vi "DSF.Engine.Plugin.Set Engine Base Pointer.vi"(8 "error in (no error)":errorcluster, 10 "Engine Base Pointer":refnum<class "DSF.Engine.Pointer.DBL.lvclass">, 11 "Plugin in":refnum<class "DSF.Engine.Plugin.lvclass">) -> (0 "error out":errorcluster, 3 "Plugin out":refnum<class "DSF.Engine.Plugin.lvclass">)   [LabVIEW 2017, in "DSF.Engine.lvlib" / "DSF.Engine.Plugin.lvclass"]
uses:
  DSF.Engine.Plugin.lvclass
  Pointer/DSF.Engine.Pointer.DBL.lvclass
  DSF.Engine.Plugin.lvclass/DSF.Engine.Plugin.ctl
  Transfer/DSF.Engine.Transfer Group.lvclass
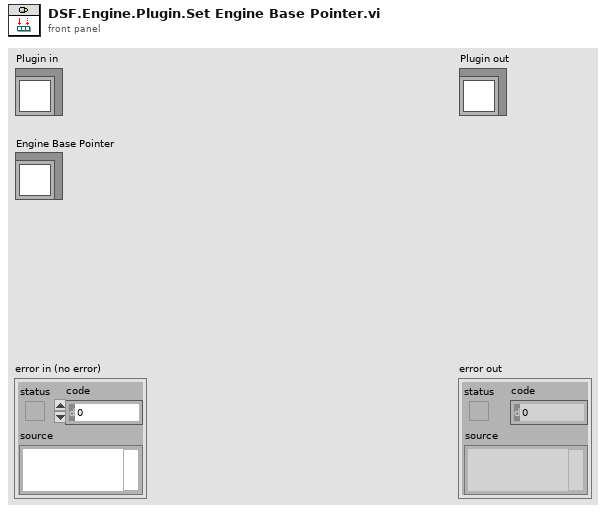
[diagram p1: front panel]
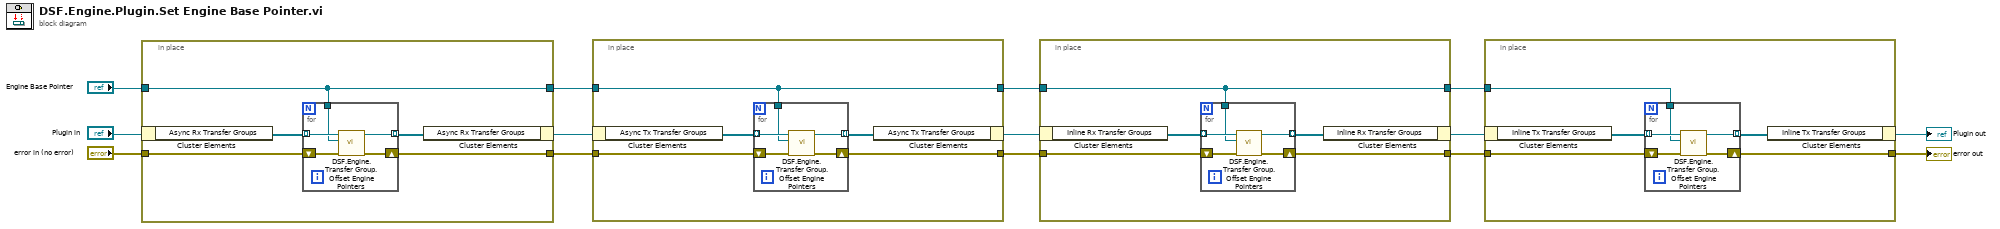
[diagram p0: block diagram]
diagram:
  n1 = in-place {
    in-place-border: "error in (no error)" -> [w17]
    in-place-border: "Engine Base Pointer" -> [w15]
    in-place-border: [w16] -> w10
    in-place-border: [w15] -> w9
    n2 = in-place-cluster #1("Plugin in") -> ("Async Rx Transfer Groups"=w19:refnum<class "DSF.Engine.Transfer Group.lvclass">[])
    n3 = for {
      tunnel: w19 -> [w24] mode=indexing
      tunnel: [w23] -> w18 mode=indexing
      shift-right: [w22] -> w16
      shift-left: w17 -> [w21]
      tunnel: w15 -> [w20]
      n4 = call "DSF.Engine.Transfer Group.Offset Engine Pointers.vi"("error in (no error)"=w21, "engine base Pointer"=w20, "Transfer Group in"=w24) -> ("error out"=w22:errorcluster, "Transfer Group out"=w23:refnum<class "DSF.Engine.Transfer Group.lvclass">)  [unwired: 7 in]
    }
    n5 = in-place-cluster #1("Async Rx Transfer Groups"=w18) -> (w11:refnum<class "DSF.Engine.Plugin.lvclass">)
  }
  n6 = in-place {
    in-place-border: w10 -> [w27]
    in-place-border: w9 -> [w25]
    in-place-border: [w26] -> w7
    in-place-border: [w25] -> w6
    n7 = in-place-cluster #2(w11) -> ("Async Tx Transfer Groups"=w29:refnum<class "DSF.Engine.Transfer Group.lvclass">[])
    n8 = for {
      tunnel: w29 -> [w34] mode=indexing
      tunnel: [w33] -> w28 mode=indexing
      shift-right: [w32] -> w26
      shift-left: w27 -> [w31]
      tunnel: w25 -> [w30]
      n9 = call "DSF.Engine.Transfer Group.Offset Engine Pointers.vi"("error in (no error)"=w31, "engine base Pointer"=w30, "Transfer Group in"=w34) -> ("error out"=w32:errorcluster, "Transfer Group out"=w33:refnum<class "DSF.Engine.Transfer Group.lvclass">)  [unwired: 7 in]
    }
    n10 = in-place-cluster #2("Async Tx Transfer Groups"=w28) -> (w8:refnum<class "DSF.Engine.Plugin.lvclass">)
  }
  n11 = in-place {
    in-place-border: w7 -> [w37]
    in-place-border: w6 -> [w35]
    in-place-border: [w36] -> w4
    in-place-border: [w35] -> w3
    n12 = in-place-cluster #3(w8) -> ("Inline Rx Transfer Groups"=w39:refnum<class "DSF.Engine.Transfer Group.lvclass">[])
    n13 = for {
      tunnel: w39 -> [w44] mode=indexing
      tunnel: [w43] -> w38 mode=indexing
      shift-right: [w42] -> w36
      shift-left: w37 -> [w41]
      tunnel: w35 -> [w40]
      n14 = call "DSF.Engine.Transfer Group.Offset Engine Pointers.vi"("error in (no error)"=w41, "engine base Pointer"=w40, "Transfer Group in"=w44) -> ("error out"=w42:errorcluster, "Transfer Group out"=w43:refnum<class "DSF.Engine.Transfer Group.lvclass">)  [unwired: 7 in]
    }
    n15 = in-place-cluster #3("Inline Rx Transfer Groups"=w38) -> (w5:refnum<class "DSF.Engine.Plugin.lvclass">)
  }
  n16 = in-place {
    in-place-border: w4 -> [w46]
    in-place-border: w3 -> [w47]
    in-place-border: [w45] -> w1
    n17 = in-place-cluster #4(w5) -> ("Inline Tx Transfer Groups"=w49:refnum<class "DSF.Engine.Transfer Group.lvclass">[])
    n18 = for {
      tunnel: w49 -> [w54] mode=indexing
      tunnel: [w53] -> w48 mode=indexing
      shift-right: [w52] -> w45
      shift-left: w46 -> [w51]
      tunnel: w47 -> [w50]
      n19 = call "DSF.Engine.Transfer Group.Offset Engine Pointers.vi"("error in (no error)"=w51, "engine base Pointer"=w50, "Transfer Group in"=w54) -> ("error out"=w52:errorcluster, "Transfer Group out"=w53:refnum<class "DSF.Engine.Transfer Group.lvclass">)  [unwired: 7 in]
    }
    n20 = in-place-cluster #4("Inline Tx Transfer Groups"=w48) -> (→"Plugin out":refnum<class "DSF.Engine.Plugin.lvclass">)
  }
  "error out" <- w1
